vi "SERVOSETTING.vi"   [LabVIEW 2016, in "Test2.lvrbt"]
uses:
  Test2.lvrbt
  <vilib>/NXT/Hardware/Plugins/Tetrix 180 deg Servo/Tetrix180ServoAddress.ctl
  <vilib>/NXT/NXTIO Xnodes/NXTIONodeSubVIs/TETRIX IO Move Servos.vi
  <vilib>/NXT/Dual Mode Library/Waits/Wait_Num.vi
  <vilib>/NXT/NXTIO Xnodes/AddressXNode/NXTIOAddress.xnode
  <vilib>/NXT/Subs/LVHSConnector.ctl
  <vilib>/NXT/NXTIO Xnodes/NXTIOXNode/NXTIO.xnode
  <vilib>/NXT/LegoClasses/BrickReference/BrickReference.lvclass
types:
  T1 = typedef "Tetrix180ServoAddress.ctl" = i32
  T2 = cluster{"Tetrix180Servo":T1, "Tetrix180Servo":T1, "Tetrix180Servo":T1, "Tetrix180Servo":T1, "Tetrix180Servo":T1, "Tetrix180Servo":T1}
  T3 = typedef "LVHSConnector.ctl" = refnum<class "BrickReference.lvclass">
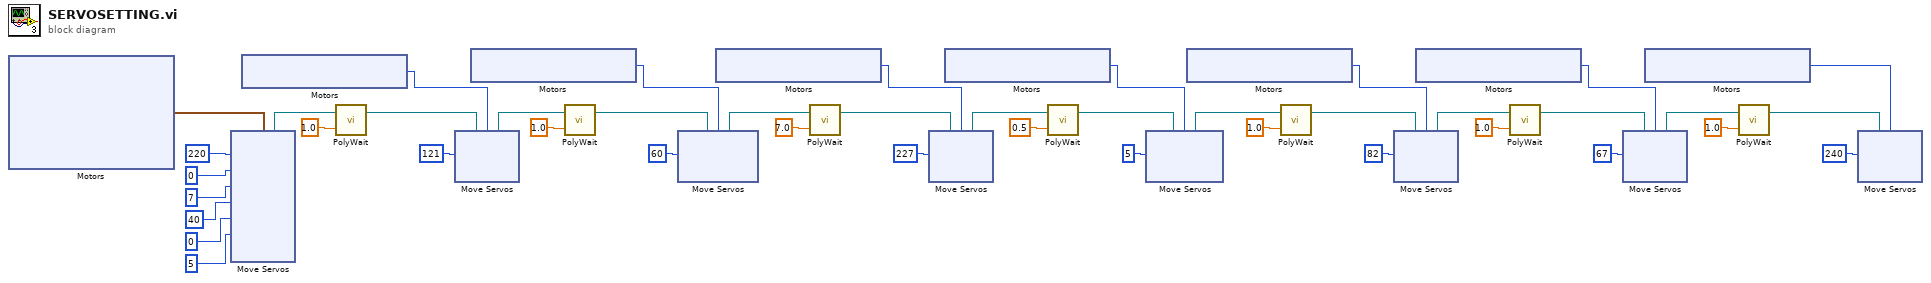
[diagram p0: block diagram]
diagram:
  n1 = xnode "Motors"() -> ("Motor"=w30:T2)
  n2 = xnode "Move Servos"("Position 6"=u8 5, "Position 5"=u8 0, "Position 4"=u8 40, "Position 3"=u8 7, "Position 2"=u8 0, "Position 1"=u8 220, "Motors"=w30) -> ("NXT/EV3"=w7:T3)  [unwired: 1 in]
  n3 = xnode "Motors"() -> ("Motor"=w6:T1)
  n4 = call-poly <vilib>:"PolyWait.vi"("Time (1 sec)"=sgl 1.0, "NXT/EV3"=w7) -> ("NXT/EV3"=w2:T3)  [unwired: 2 in]
  n5 = xnode "Move Servos"("Position 1"=u8 121, "Motors"=w6, "NXT/EV3"=w2) -> ("NXT/EV3"=w4:T3)
  n6 = xnode "Motors"() -> ("Motor"=w42:T1)
  n7 = call-poly <vilib>:"PolyWait.vi"("Time (1 sec)"=sgl 1.0, "NXT/EV3"=w4) -> ("NXT/EV3"=w18:T3)  [unwired: 2 in]
  n8 = xnode "Move Servos"("Position 1"=u8 60, "Motors"=w42, "NXT/EV3"=w18) -> ("NXT/EV3"=w39:T3)
  n9 = xnode "Motors"() -> ("Motor"=w38:T1)
  n10 = call-poly <vilib>:"PolyWait.vi"("Time (1 sec)"=sgl 7.0, "NXT/EV3"=w39) -> ("NXT/EV3"=w36:T3)  [unwired: 2 in]
  n11 = xnode "Move Servos"("Position 1"=u8 227, "Motors"=w38, "NXT/EV3"=w36) -> ("NXT/EV3"=w34:T3)
  n12 = xnode "Motors"() -> ("Motor"=w33:T1)
  n13 = call-poly <vilib>:"PolyWait.vi"("Time (1 sec)"=sgl 0.5, "NXT/EV3"=w34) -> ("NXT/EV3"=w31:T3)  [unwired: 2 in]
  n14 = xnode "Move Servos"("Position 1"=u8 5, "Motors"=w33, "NXT/EV3"=w31) -> ("NXT/EV3"=w23:T3)
  n15 = xnode "Motors"() -> ("Motor"=w21:T1)
  n16 = call-poly <vilib>:"PolyWait.vi"("Time (1 sec)"=sgl 1.0, "NXT/EV3"=w23) -> ("NXT/EV3"=w20:T3)  [unwired: 2 in]
  n17 = xnode "Move Servos"("Position 1"=u8 82, "Motors"=w21, "NXT/EV3"=w20) -> ("NXT/EV3"=w1:T3)
  n18 = xnode "Motors"() -> ("Motor"=w15:T1)
  n19 = call-poly <vilib>:"PolyWait.vi"("Time (1 sec)"=sgl 1.0, "NXT/EV3"=w1) -> ("NXT/EV3"=w14:T3)  [unwired: 2 in]
  n20 = xnode "Move Servos"("Position 1"=u8 67, "Motors"=w15, "NXT/EV3"=w14) -> ("NXT/EV3"=w12:T3)
  n21 = xnode "Motors"() -> ("Motor"=w10:T1)
  n22 = call-poly <vilib>:"PolyWait.vi"("Time (1 sec)"=sgl 1.0, "NXT/EV3"=w12) -> ("NXT/EV3"=w9:T3)  [unwired: 2 in]
  n23 = xnode "Move Servos"("Position 1"=u8 240, "Motors"=w10, "NXT/EV3"=w9) -> ()  [unwired: 1 out]
